vi "GetIconName.vi"(0 "Library":refnum<vi>, 2 "VI name":string, 5 "error in":errorcluster) -> (14 "FP title":string, 16 "MethodName":string, 19 "error out":errorcluster)   [LabVIEW 2017, in "G#IDE.lvlib" / "IconLib.lvlib"]
uses:
  <resource>/Framework/Providers/AddQ/G#IDE/support/IconLib/IconLib.lvlib
  <vilib>/regexp/Match Regular Expression.xnode
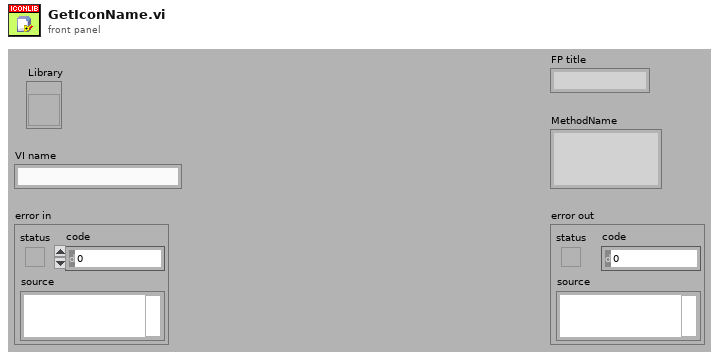
[diagram p1: front panel]
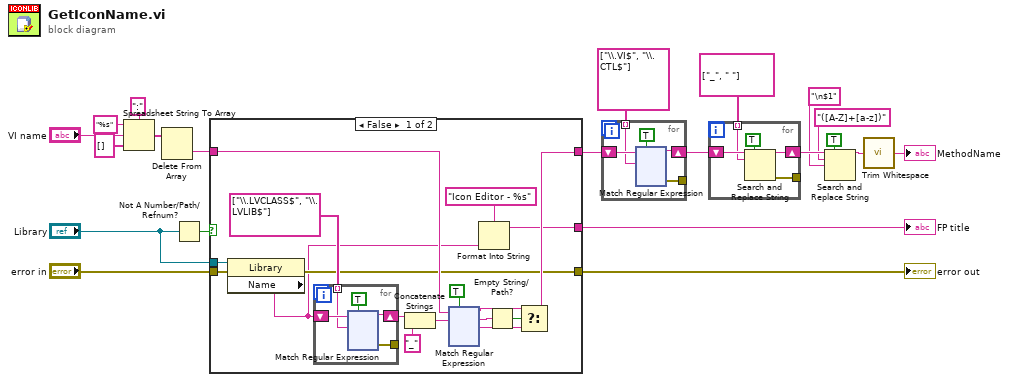
[diagram p0: block diagram]
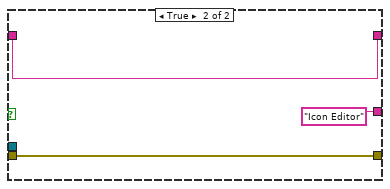
[diagram p2: hidden frame]
diagram:
  n1 = Spreadsheet String To Array(delimiter (Tab)=":", format string="%s", spreadsheet string="VI name", array type (2D Dbl)=string[] []) -> (array=w19:string[])
  n2 = Delete From Array(array=w19) -> (deleted portion=w9:string)  [unwired: 2 in, 1 out]
  n3 = Not A Number/Path/Refnum?(number/path/refnum="Library") -> (NaN/Path/Refnum?=w5:bool)
  n4 = case shown="False" w5 {
    tunnel: "error in" -> [w38 w268]
    tunnel: "Library" -> [w37 _]
    tunnel: [w26 w268] -> w6
    tunnel: w9 -> [w32 w267]
    tunnel: [w27 w267] -> w8
    tunnel: [w22 "Icon Editor"] -> w1
    frame False {
      n5 = property class="Library"(reference=w37, error in=w38) -> (error out=w26:errorcluster, "Name"=w23:string)  [unwired: 1 out]
      n6 = for {
        tunnel: [w153] -> _
        shift-right: [w151] -> w35
        shift-left: w23 -> [w152]
        tunnel: string[] ["\\.LVCLASS$", "\\.LVLIB$"] -> [w150] mode=indexing
        n7 = xnode "Match Regular Expression"("input string"=w152, "regular expression"=w150, "ignore case? (F)"=TRUE) -> ("before match"=w151:string, "error out"=w153:errorcluster)  [unwired: 3 in, 3 out]
      }
      n8 = Concatenate Strings(w35, "_" ("string")) -> (w33:string)
      n9 = xnode "Match Regular Expression"("input string"=w32, "regular expression"=w33, "ignore case? (F)"=TRUE) -> ("before match"=w28:string, "whole match"=w31:string, "after match"=w29:string)  [unwired: 3 in, 2 out]
      n10 = Format Into String(format string="Icon Editor - %s", w23) -> (resulting string=w22:string)  [unwired: 2 in, 1 out]
      n11 = Empty String/Path?(string/path=w31) -> (empty?=w30:bool)
      n12 = Select(t=w28, s=w30, f=w29) -> (s? t:f=w27:string)
    }
    frame True {
    }
  }
  "error out" <- w6
  "FP title" <- w1
  n13 = for {
    tunnel: [w272] -> _
    shift-right: [w270] -> w12
    shift-left: w8 -> [w271]
    tunnel: string[] ["\\.VI$", "\\.CTL$"] -> [w269] mode=indexing
    n14 = xnode "Match Regular Expression"("input string"=w271, "regular expression"=w269, "ignore case? (F)"=TRUE) -> ("before match"=w270:string, "error out"=w272:errorcluster)  [unwired: 3 in, 3 out]
  }
  n15 = for {
    shift-right: [w389] -> w17
    shift-left: w12 -> [w387]
    tunnel: string[] ["_", " "] -> [w386] mode=indexing
    tunnel: [w385] -> _
    n16 = Search and Replace String(replace all?=TRUE ("replace all? (F)"), input string=w387, search string=w386) -> (result string=w389:string, error out=w385:errorcluster)  [unwired: 2 in, 5 out]
  }
  n17 = Search and Replace String(replace all?=TRUE ("replace all? (F)"), input string=w17, search string="([A-Z]+[a-z])", replace string="\n$1" ("replace string (\"\")")) -> (result string=w14:string)  [unwired: 1 in, 6 out]
  n18 = call <vilib>:"Trim Whitespace.vi"("string"=w14) -> ("trimmed string"=→"MethodName":string)  [unwired: 1 in]
